vi "Do.vi"(8 "error in (no error)":errorcluster, 10 "Actor in":refnum<class "Actor.lvclass">, 11 "ReadData Msg":refnum<class "ReadData Msg.lvclass">) -> (0 "error out":errorcluster, 2 "Actor out":refnum<class "Actor.lvclass">)   [LabVIEW 2025, in "PLC_Module.lvlib" / "ReadData Msg.lvclass"]
doc: "This VI delivers the message to the actor by calling the appropriate method(s) on the actor."
uses:
  ReadData Msg.lvclass
  <vilib>/ActorFramework/Actor/Actor.lvclass
  ReadData Msg.lvclass/ReadData Msg.ctl
  PLC_Module/PLC_Module.lvclass
  9ef47adc-f318-494c-9b8b-6df3216d6863.vi
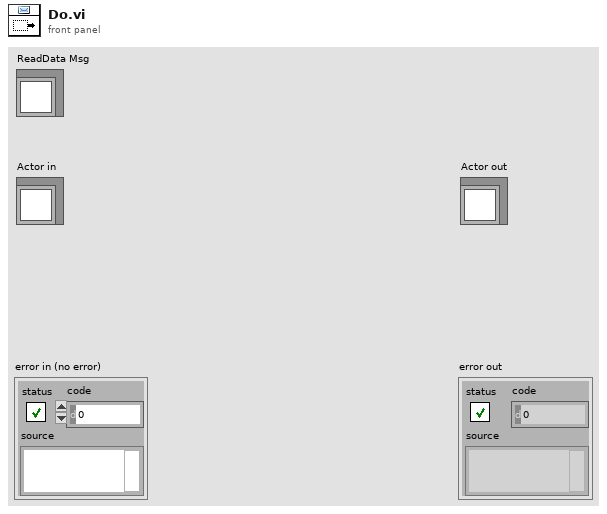
[diagram p1: front panel]
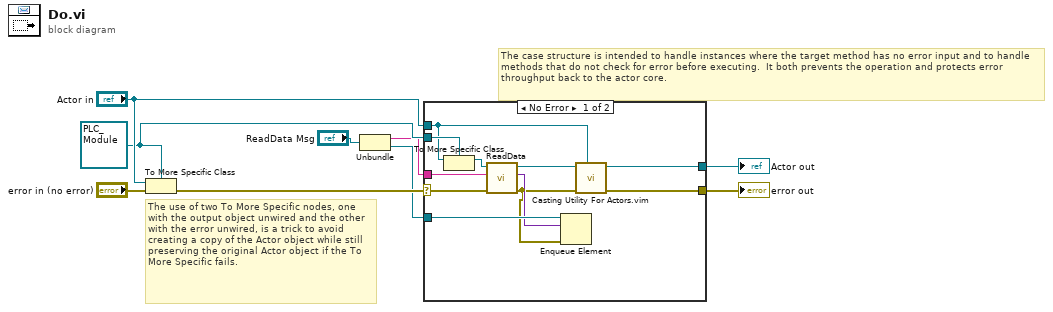
[diagram p0: block diagram]
diagram:
  w3 = refnum<class "PLC_Module.lvclass"> refnum ("Actor in")
  # "The use of two To More Specific nodes, one with the output object unwired and the other with the error unwired, is a trick to avoid creating a copy of the Actor object while still preserving the original Actor object if the To More Specific fails."
  # "The case structure is intended to handle instances where the target method has no error input and to handle methods that do not check for error before executing.  It both prevents the operation and protects error throughput back to the actor core."
  n1 = To More Specific Class(target class=w3, reference="Actor in", error in="error in (no error)") -> (error out=w7:errorcluster)  [unwired: 1 out]
  n2 = Unbundle("ReadData Msg") -> (w2:string, w1:refnum<queue>)
  n3 = case shown="No Error" w7 {
    selector: w7 -> [w20 w22]
    tunnel: [w14 w22] -> w6
    tunnel: [w15 w21] -> w5
    tunnel: "Actor in" -> [w17 w21]
    tunnel: w3 -> [w18 _]
    tunnel: w2 -> [w13 _]
    tunnel: w1 -> [w12 _]
    frame No Error {
      n4 = To More Specific Class(target class=w18, reference=w17) -> (specific class reference=w19:refnum<class "PLC_Module.lvclass">)  [unwired: 1 in, 1 out]
      n5 = call "ReadData.vi"("error in (no error)"=w20, "LogicName"=w13, "PLC_Module in"=w19) -> ("error out"=w10:errorcluster, "Data"=w11:variant, "PLC_Module out"=w16:refnum<class "PLC_Module.lvclass">)  [unwired: 6 in]
      n6 = Enqueue Element(queue=w12, element=w11, error in (no error)=w10) -> ()  [unwired: 1 in, 3 out]
      n7 = call "Casting Utility For Actors.vim"("type"=w17, "error in (no error)"=w10, "Actor in"=w16) -> ("error out"=w14:errorcluster, "Actor out"=w15:refnum<class "Actor.lvclass">)  [unwired: 7 in]
    }
    frame Error {
      # "If type check fails, pass the original object out again."
    }
  }
  "error out" <- w6
  "Actor out" <- w5
